vi "Bug Detect.vi"(3 "Frequency of Wood (in KHz)":dbl) -> (0 "Signal":dynamicdata(graph), 1 "Filtered signal":dynamicdata(graph), 2 "Bug Detected":bool)   [LabVIEW 2019]
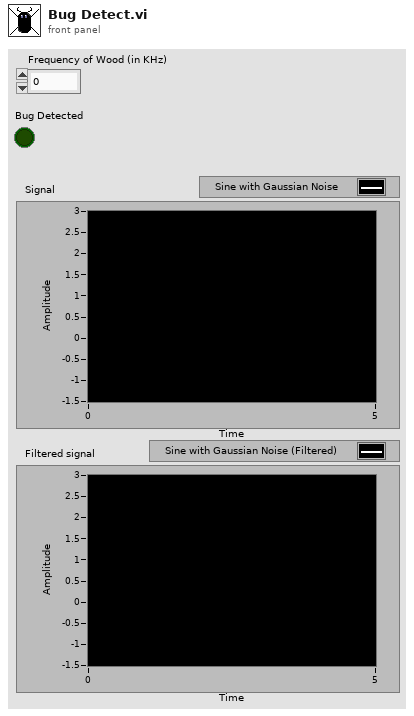
[diagram p1: front panel]
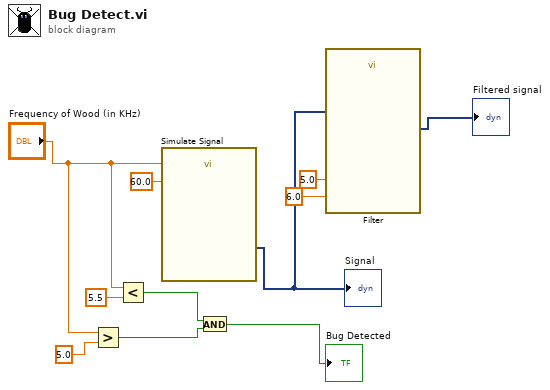
[diagram p0: block diagram]
diagram:
  n1 = Greater?(x="Frequency of Wood (in KHz)", y=5.0) -> (0:w6:bool)
  n2 = Less?(x="Frequency of Wood (in KHz)", y=5.5) -> (x < y?=w7:bool)
  n3 = call "Simulate Signal"("Frequency"="Frequency of Wood (in KHz)", "Phase"=60.0) -> ("Sine with Gaussian Noise"=w4:dynamicdata)  [unwired: 12 in, 1 out]
  "Signal" <- w4
  n4 = And(x=w7, y=w6) -> (x .and. y?=→"Bug Detected":bool)
  n5 = call "Filter"("Lower Cut-Off"=5.0, "Upper Cut-Off"=6.0, "Signal"=w4) -> ("Filtered Signal"=→"Filtered signal":dynamicdata)  [unwired: 7 in, 1 out]
